vi "Network - Send DS eventstring.vi"(8 "error in":errorcluster, 10 "URL":string="127.0.0.1", 11 "Numeric":dbl) -> (0 "error out":errorcluster)   [LabVIEW 2009, in "Core SubVIs.lvlib"]
uses:
  Core SubVIs.lvlib
panel:
  out "Connected":bool
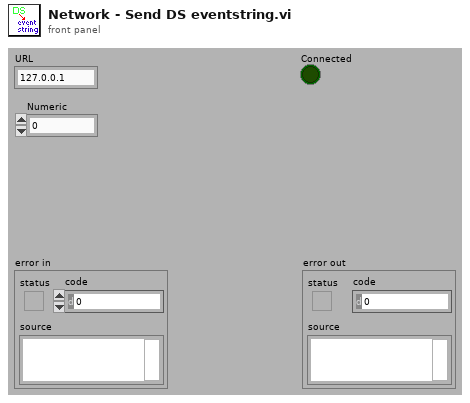
[diagram p1: front panel]
types:
  T1 = enum16{"Read", "Write", "ReadWrite", "BufferedRead", "BufferedReadWrite"}
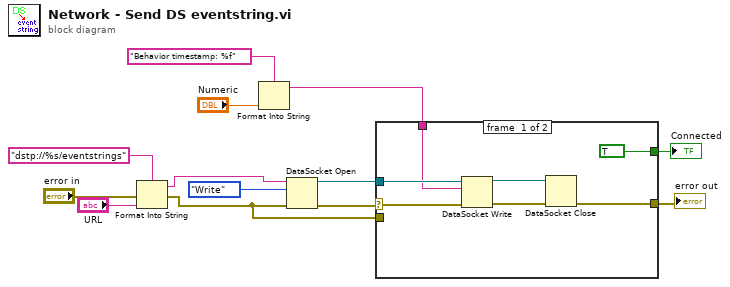
[diagram p0: block diagram]
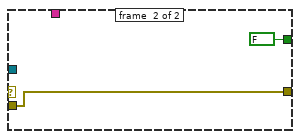
[diagram p2: hidden frame]
diagram:
  n1 = Format Into String(format string="dstp://%s/eventstrings", error in="error in", "URL") -> (resulting string=w9:string, error out=w1:errorcluster)  [unwired: 1 in]
  n2 = Format Into String(format string="Behavior timestamp: %f", "Numeric") -> (resulting string=w2:string)  [unwired: 2 in, 1 out]
  n3 = DataSocket Open(8:w1, 10:T1."Write" ("mode"), 11:w9) -> (0:w7:errorcluster, 3:w13:refnum<k13>)  [unwired: 1 out]
  n4 = case shown="Error" w7 {
    selector: w7 -> [w17 _]
    tunnel: w13 -> [w20 _]
    tunnel: [w16 w21] -> w6
    tunnel: [TRUE FALSE] -> w5
    tunnel: w2 -> [w14 _]
    tunnel: w1 -> [_ w21]
    frame #0 {
      n5 = DataSocket Write(8:w17, 10:w14, 11:w20) -> (0:w19:errorcluster, 3:w18:refnum<k13>)  [unwired: 2 out]
      n6 = DataSocket Close(8:w19, 11:w18) -> (0:w16:errorcluster)  [unwired: 2 out]
    }
    frame #1 {
    }
  }
  "error out" <- w6
  "Connected" <- w5
